vi "RichToFlatcif_manager_QueryTypeSettings.vi"(5 "OutputClusterType":T1, 11 "InputCluster":T2) -> (3 "OutputCluster":T1)   [LabVIEW 2021, in "CIF_PluginLoader_server.lvlib"]
uses:
  CIF_PluginLoader_server.lvlib
  cif_manager_QueryTypeSettings.ctl
  cif_manager_QueryTypeSettings_Flat.ctl
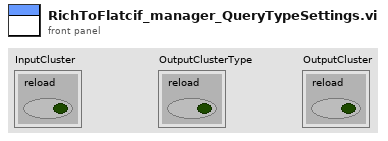
[diagram p1: front panel]
types:
  T1 = typedef "CIF_PluginLoader_server.lvlib/cif_manager_QueryTypeSettings_Flat.ctl" = cluster{"reload":bool}
  T2 = typedef "CIF_PluginLoader_server.lvlib/cif_manager_QueryTypeSettings.ctl" = cluster{"reload":bool}
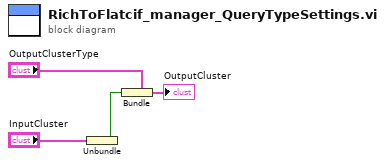
[diagram p0: block diagram]
diagram:
  n1 = Unbundle "Unbundle"("InputCluster") -> ("reload"=w1:bool)
  n2 = Bundle "Bundle"(cluster="OutputClusterType", "reload"=w1) -> (→"OutputCluster":T1)
